vi "Serialize Data.vi"(8 "error in (no error)":errorcluster, 11 "Process Data":T1 {"LIN Frame Array"."event ID" format="%x"; "LIN Frame Array"."payload" format="%x"; "LIN Frame Array"."timestamp" format="%<%.7X\n%x>T"; "LIN Frame Array"."type" items=["LIN Data"=64, "LIN Bus Error"=65, "LIN No Response"=66, "Delay"=224, "Log Trigger"=225, "Start Trigger"=226]; "LIN Frame Array"."identifier" format="%x"}) -> (0 "error out":errorcluster, 3 "Flat Data out":string)   [LabVIEW 2020, in "LIN Frame Array.lvlib"]
doc: "Version 0.1"
uses:
  <vilib>/ADAS Record/CustomDataTypes/LIN Frame Array/Process Data.ctl
  <vilib>/ADAS Record/CustomDataTypes/LIN Frame Array/LIN Frame.ctl
  <vilib>/ADAS Record/IODataPEF/CfgMgr/FlatFormat.ctl
  69b4f655-d322-486f-8d65-ee31f7d8c6ef.vi
  <vilib>/ADAS Record/IODataPEF/Error/Error_CheckAndSetDllError.vi
  <vilib>/ADAS Record/IODataPEF/Error/Error_SetError.vi
  <vilib>/ADAS Record/IODataPEF/CfgMgr/GetPEFConfiguration_DefaultFlatFormat.vi
  <vilib>/ADAS Record/IODataPEF/Error/ErrorMgr.vi
  <vilib>/ADAS Record/CustomData/_Custom_RegisterType.vi
  <vilib>/ADAS Record/CustomDataTypes/LIN Frame Array/LIN Frame Array.lvlib
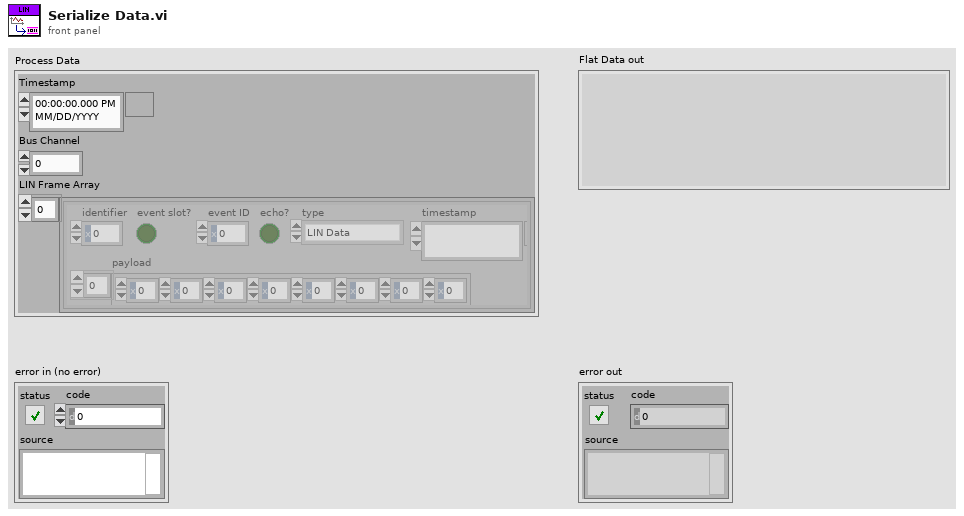
[diagram p1: front panel]
types:
  T1 = typedef "LIN Frame Array.lvlib/Process Data.ctl" = cluster{"Timestamp":timestamp, "Bus Channel":u16, "LIN Frame Array":T2[]}
  T2 = typedef "LIN Frame Array.lvlib/LIN Frame.ctl" = cluster{"timestamp":timestamp, "payload":u8[], "identifier":u32, "type":u8, "event ID":u8, "event slot?":bool, "echo?":bool}
  T3 = typedef "FlatFormat.ctl" = enum32{"Auto", "PEF", "GFB (Apache)", "GFB", "JSON", "Readable JSON", "LV String", "Reserved", "LV Native"}
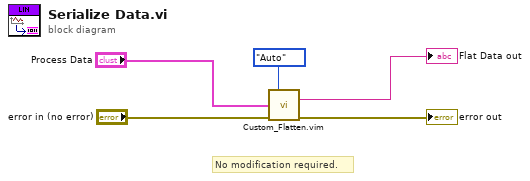
[diagram p0: block diagram]
diagram:
  # "No modification required."
  n1 = call "Custom_Flatten.vim"("Flat Format"=FlatFormat."Auto", "Data"="Process Data", "error in (no error)"="error in (no error)") -> ("Flat Data"=→"Flat Data out":string, "Error (out)"=→"error out":errorcluster)  [unwired: 10 in, 1 out]
